vi "Pockels Cal-Conditions entry window.vi"(7 "Colour":u32(colorbox)=16777225, 8 "error in (no error)":errorcluster, 10 "Update existing file":bool) -> (0 "error out":errorcluster, 1 "Cancelled (Left button pressed)":bool)   [LabVIEW 2020]
doc: "Use this template to create a dialog box with event handling."
uses:
  <vilib>/Utility/miscctls.llb/LVPointTypeDef.ctl
  Globals/gl_Calibration globals.vi
  Global Variables/General Globals.vi
panel:
  in  "Laser power":u16=2039
  in  "Pockels bias":i16=199
  in  "Prism-2":u16=1953
  in  "Prism-1":u16=2039
  in  "Cancel":bool
  in  "OK":bool
  out "Message":string="IMPORTANT!\n\nEnter the current settings of pre-chirper prism positions, the bias setting shown on the Pockels controller unit, and the laser power shown on the laser controller.\n\nNote: These values will be stored in the pockels calibration file and used each time a new calibration curve is about to be added in order to verify rig setup validity, to ensure the calibration file remains valid.\n"
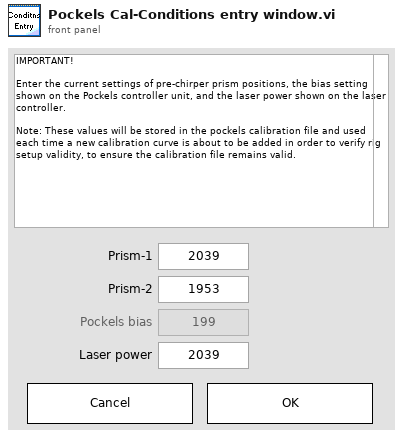
[diagram p1: front panel]
types:
  T1 = typedef "LVPointTypeDef.ctl" = cluster{"Horizontal":i16, "Vertical":i16}
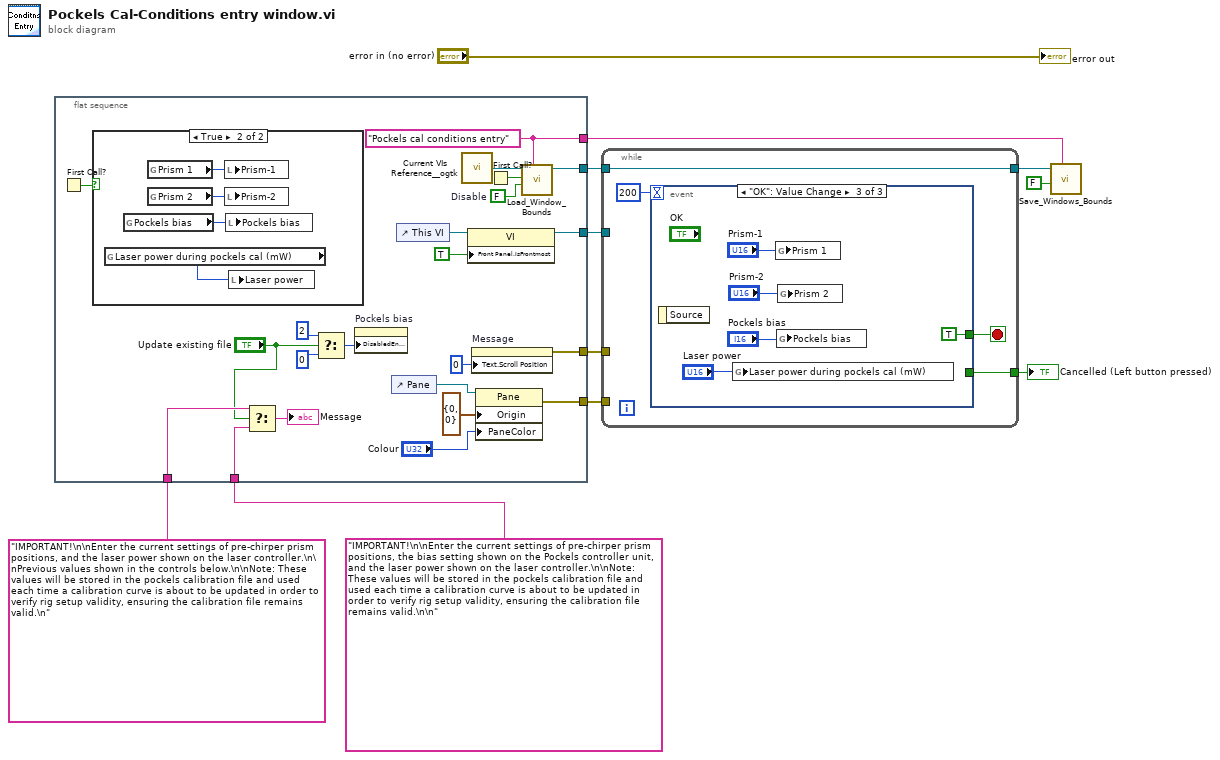
[diagram p0: block diagram]
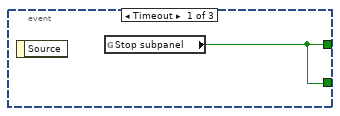
[diagram p3: hidden frame]
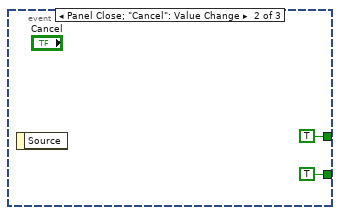
[diagram p4: hidden frame]
diagram:
  n1 = flat-sequence {
    tunnel: [w32] -> w11
    tunnel: [w29] -> w10
    tunnel: [w27] -> w9
    tunnel: [w22] -> w7
    tunnel: [w21] -> w5
    tunnel: "IMPORTANT!\n\nEnter the current settings of pre-chirper prism positions, the bias setting shown on the Pockels controller unit, and the laser power shown on the laser controller.\n\nNote: These values will be stored in the pockels calibration file and used each time a calibration curve is about to be updated in order to verify rig setup validity, ensuring the calibration file remains valid.\n\n" ("Message") -> [w14]
    tunnel: "IMPORTANT!\n\nEnter the current settings of pre-chirper prism positions, and the laser power shown on the laser controller.\n\nPrevious values shown in the controls below.\n\nNote: These values will be stored in the pockels calibration file and used each time a calibration curve is about to be updated in order to verify rig setup validity, ensuring the calibration file remains valid.\n" ("Message") -> [w13]
    frame #0 {
      w23 = FALSE  # Disable
      w22 = "Pockels cal conditions entry" ("Window Name (i.e. Key)")
      n2 = First Call?() -> (First Call?: T/F=w19:bool)
      n3 = case shown="True" w19 {
        frame False {
        }
        frame True {
          n4 = global read "gl_Calibration globals.vi" "Laser power during pockels cal (mW)"() -> (w34:u16)
          n5 = global read "gl_Calibration globals.vi" "Pockels bias"() -> (w35:i16)
          n6 = global read "gl_Calibration globals.vi" "Prism 1"() -> (w37:u16)
          n7 = global read "gl_Calibration globals.vi" "Prism 2"() -> (w36:u16)
          n8 = local write "Prism-1"(w37) -> ()
          n9 = local write "Prism-2"(w36) -> ()
          n10 = local write "Pockels bias"(w35) -> ()
          n11 = local write "Laser power"(w34) -> ()
        }
      }
      n12 = Select(t=w13, s="Update existing file", f=w14) -> (s? t:f=→"Message":string)
      n13 = Select(t=2, s="Update existing file", f=0) -> (s? t:f=w18:i32)
      n14 = property on="Pockels bias" class="DigNum (strict)"("DisabledEnum"=w18) -> ()  [unwired: 2 in, 2 out]
      n15 = control-ref of="Pane"() -> (w26:refnum<vi>)
      n16 = control-ref of="This VI"() -> (w30:refnum<vi>)
      n17 = call <userlib>:"Current VIs Reference__ogtk.vi"() -> ("Current VI's reference"=w25:refnum<vi>)  [unwired: 5 in]
      n18 = property on="Property Node" class="VI"(reference=w30, "Front Panel.IsFrontmost"=TRUE ("Front Panel Window:Is Frontmost")) -> (reference out=w29:refnum<vi>)  [unwired: 1 in, 1 out]
      n19 = property on="Message" class="Str"("Text.Scroll Position"=u32 0) -> (error out=w32:errorcluster)  [unwired: 2 in, 1 out]
      n20 = property class="Pane"(reference=w26, "Origin"=T1 {"Horizontal"=0, "Vertical"=0}, "PaneColor"="Colour") -> (error out=w27:errorcluster)  [unwired: 1 in, 1 out]
      n21 = First Call?() -> (First Call?: T/F=w24:bool)
      n22 = call "Load_Window_Bounds.vi"("Window Name (i.e. Key)"=w22, "Disable"=w23, "First Call"=w24, "Window VI's Ref"=w25) -> ("reference out"=w21:refnum<vi>)  [unwired: 4 in, 3 out]
    }
  }
  n23 = while {
    tunnel: w11 -> [_]
    tunnel: w9 -> [_]
    tunnel: w10 -> [_]
    tunnel: [w39] -> w8
    tunnel: w5 -> [w38]
    tunnel: [w38] -> w4
    stop <- w41 stop-if-true
    n24 = event shown="[2] \"OK\": Value Change" {
      selector: _ -> [_ _ _]
      dyn-events: _ -> [_ _ _]
      timeout: 200 -> [_ _ _]
      tunnel: [w42 TRUE ("Stop?") TRUE ("Stop?")] -> w41
      tunnel: [w42 TRUE ("Stop subpanel") _] -> w39
      event Timeout {
        n25 = event-data() -> ()  [unwired: 1 in, 1 out]
        n26 = global read "General Globals.vi" "Stop subpanel"() -> (w42:bool)
      }
      event Panel Close; "Cancel": Value Change {
        n27 = event-data() -> ()  [unwired: 1 in, 1 out]
      }
      event "OK": Value Change {
        n28 = event-data() -> ()  [unwired: 1 in, 1 out]
        n29 = global write "gl_Calibration globals.vi" "Laser power during pockels cal (mW)"("Laser power") -> ()
        n30 = global write "gl_Calibration globals.vi" "Prism 1"("Prism-1") -> ()
        n31 = global write "gl_Calibration globals.vi" "Pockels bias"("Pockels bias") -> ()
        n32 = global write "gl_Calibration globals.vi" "Prism 2"("Prism-2") -> ()
      }
    }
  }
  "Cancelled (Left button pressed)" <- w8
  n33 = call "Save_Windows_Bounds.vi"("Window Name (i.e. Key)"=w7, "Front Panel Window:Open"=FALSE, "Window VI's Ref"=w4) -> ()  [unwired: 8 in, 1 out]
  "error out" <- "error in (no error)"
